vi "BuildKey.vi"(8 "error in (no error)":errorcluster, 9 "Column (65=A)":i32=65, 10 "Row (>=1)":i32=1, 11 "object in":refnum<class "Piece.lvclass">) -> (0 "error out":errorcluster, 2 "Built Key":map{string, i32}(c390), 3 "object out":refnum<class "Piece.lvclass">)   [LabVIEW 2020, in "Piece.lvclass"]
doc: "Builds the key for the map"
uses:
  Piece.lvclass
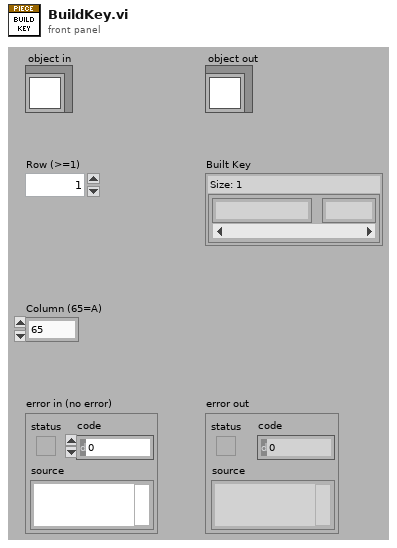
[diagram p1: front panel]
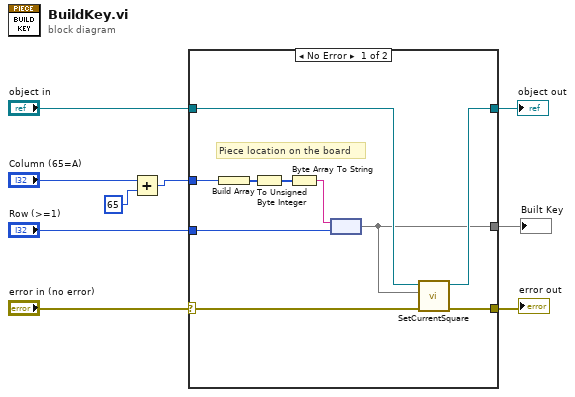
[diagram p0: block diagram]
diagram:
  n1 = Add(x="Column (65=A)", y=65) -> (x+y=w2:i32)
  n2 = case shown="No Error" "error in (no error)" {
    selector: "error in (no error)" -> [w13 w21]
    tunnel: [w12 w21] -> w8
    tunnel: [w14 w20] -> w6
    tunnel: "object in" -> [w15 w20]
    tunnel: "Row (>=1)" -> [w17 _]
    tunnel: w2 -> [w16 _]
    tunnel: [w10 _] -> w3
    frame No Error {
      # "Piece location on the board"
      n3 = Build Array(w16) -> (w18:i32[])
      n4 = To Unsigned Byte Integer(number=w18) -> (unsigned 8bit integer=w11:u8[])
      n5 = Byte Array To String(unsigned byte array=w11) -> (string=w19:string)
      n6 = node(w19, w17) -> (w10:map{string, i32})
      n7 = call "SetCurrentSquare.vi"("error in (no error)"=w13, "currentSquare"=w10, "object in"=w15) -> ("error out"=w12:errorcluster, "object out"=w14:refnum<class "Piece.lvclass">)  [unwired: 7 in]
    }
    frame Error {
    }
  }
  "error out" <- w8
  "object out" <- w6
  "Built Key" <- w3
